vi "niFpgaBFGroupLastOdd.vi"(5 "bf data in":T1 {"x_r" format="%.16g"; "x_i" format="%.16g"; "y_r" format="%.16g"; "y_i" format="%.16g"}, 7 "stage switch in":bool, 9 "tf index in":fxp<+,10,10>) -> (6 "bf data out":T1 {"x_r" format="%.16g"; "x_i" format="%.16g"; "y_r" format="%.16g"; "y_i" format="%.16g"}, 8 "stage switch out":bool)   [LabVIEW 2017]
uses:
  <vilib>/rvi/Analysis/measure/FFT/supportingXNodes/permutation/XNode/niFpgaFFTPermutation.xnode
  <vilib>/rvi/FXPMathLib/basic elements/FxpDiscreteDelay/XNode/nifxpmath_DiscreteDelay.xnode
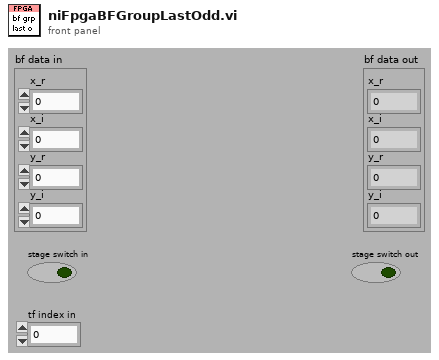
[diagram p1: front panel]
types:
  T1 = cluster{"x_r":fxp<+/-,16,1>, "x_i ":fxp<+/-,16,1>, "y_r ":fxp<+/-,16,1>, "y_i ":fxp<+/-,16,1>}
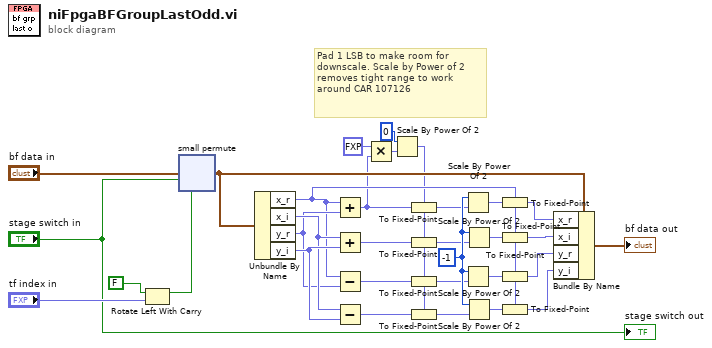
[diagram p0: block diagram]
diagram:
  w25 = -1 ("n")
  # "Pad 1 LSB to make room for\ndownscale. Scale by Power of 2 removes tight range to work around CAR 107126"
  n1 = Rotate Left With Carry(2:"tf index in", 3:FALSE ("carry")) -> (1:w28:bool)  [unwired: 1 out]
  n2 = xnode "small permute"("bf data in"="bf data in", "stage switch"="stage switch in", "perm switch"=w28) -> ("bf data out"=w15:T1)
  n3 = Unbundle By Name(w15) -> ("x_r"=w13:fxp<+/-,16,1>, "x_i"=w23:fxp<+/-,16,1>, "y_r"=w22:fxp<+/-,16,1>, "y_i"=w24:fxp<+/-,16,1>)
  n4 = Add(x=w13, y=w22) -> (x+y=w11:fxp<+/-,17,2>)
  n5 = Add(x=w23, y=w24) -> (x+y=w5:fxp<+/-,17,2>)
  n6 = Subtract(x=w13, y=w22) -> (x-y=w8:fxp<+/-,17,2>)
  n7 = Subtract(x=w23, y=w24) -> (x-y=w4:fxp<+/-,17,2>)
  n8 = Multiply(x=fxp<+,2,1> 0.0, y=w11) -> (x*y=w3:fxp<+/-,18,2>)
  n9 = Scale By Power Of 2(n=0, x=w3) -> (x*2^n=w1:fxp<+/-,18,2>)
  n10 = To Fixed-Point(fixed-point type=w1, number=w11) -> (fixed-point=w12:fxp<+/-,18,2>)
  n11 = To Fixed-Point(fixed-point type=w1, number=w5) -> (fixed-point=w9:fxp<+/-,18,2>)
  n12 = To Fixed-Point(fixed-point type=w1, number=w8) -> (fixed-point=w7:fxp<+/-,18,2>)
  n13 = To Fixed-Point(fixed-point type=w1, number=w4) -> (fixed-point=w6:fxp<+/-,18,2>)
  n14 = Scale By Power Of 2(n=w25, x=w12) -> (x*2^n=w16:fxp<+/-,18,2>)
  n15 = Scale By Power Of 2(n=w25, x=w7) -> (x*2^n=w18:fxp<+/-,18,2>)
  n16 = Scale By Power Of 2(n=w25, x=w9) -> (x*2^n=w17:fxp<+/-,18,2>)
  n17 = Scale By Power Of 2(n=w25, x=w6) -> (x*2^n=w19:fxp<+/-,18,2>)
  n18 = To Fixed-Point(fixed-point type=w13, number=w16) -> (fixed-point=w21:fxp<+/-,16,1>)
  n19 = To Fixed-Point(fixed-point type=w13, number=w17) -> (fixed-point=w20:fxp<+/-,16,1>)
  n20 = To Fixed-Point(fixed-point type=w13, number=w18) -> (fixed-point=w26:fxp<+/-,16,1>)
  n21 = To Fixed-Point(fixed-point type=w13, number=w19) -> (fixed-point=w27:fxp<+/-,16,1>)
  n22 = Bundle By Name(cluster=w15, "x_r"=w21, "x_i"=w20, "y_r"=w26, "y_i"=w27) -> (→"bf data out":T1)
  "stage switch out" <- "stage switch in"
